vi "remove channel mappings.vi"(8 "error in (no error)":errorcluster, 9 "Properties:UID":string, 10 "Channel Array":refnum<class "TBM channel.lvclass">[](array[class]), 11 "engine configuration in":refnum<class "engine configuration.lvclass">) -> (0 "error out":errorcluster, 1 "Numeric":i32, 2 "Array":string[](array[string]), 3 "engine configuration out":refnum<class "engine configuration.lvclass">, 4 "name":string, 5 "accessors:metadata":string)   [LabVIEW 2015, in "DAQmx Module editor node.lvclass"]
doc: "This VI was createde to encapsulate the multi-channel clearing of mappings on a line during configuration. \n\nThis VI became complicated when we moved to support multiple channels per line. \nWe are trying to minimize code complexity by packaging this mapping cleaning into\nthis subVI."
uses:
  DAQmx Module editor node.lvclass
  <vilib>/NI/Module Execution Interface/Engine Configuration/engine configuration.lvclass
  <vilib>/NI/Tag Bus/tag/tag descriptor.lvclass
  <vilib>/NI/Tag Bus Module Framework/channel/TBM channel.lvclass
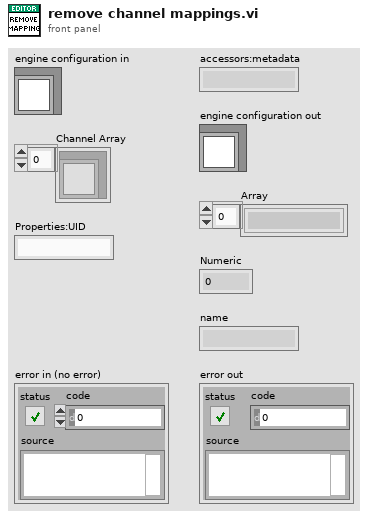
[diagram p1: front panel]
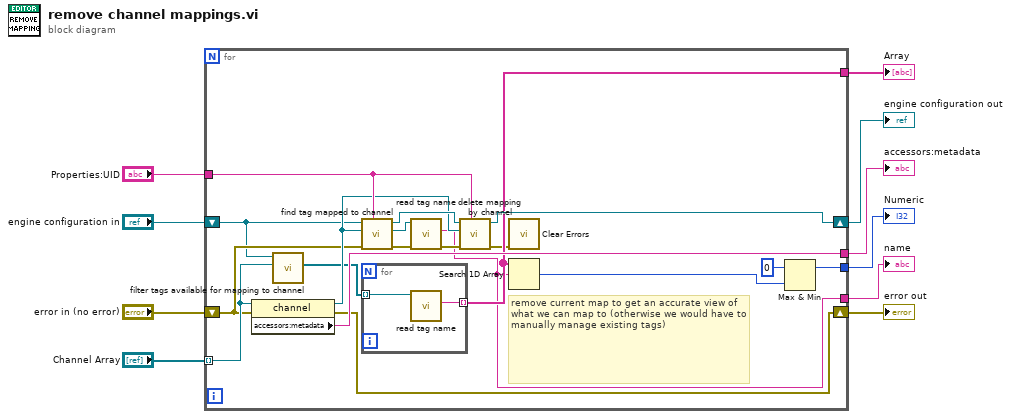
[diagram p0: block diagram]
diagram:
  n1 = for {
    tunnel: [w28] -> w2
    tunnel: "Properties:UID" -> [w27]
    tunnel: "Channel Array" -> [w19] mode=indexing
    tunnel: [w18] -> w6
    tunnel: [w14] -> w7
    tunnel: [w13] -> w8
    shift-right: [w25] -> w4
    shift-left: "error in (no error)" -> [w12]
    shift-right: [w29] -> w1
    shift-left: "engine configuration in" -> [w11]
    # "remove current map to get an accurate view of what we can map to (otherwise we would have to manually manage existing tags)"
    n2 = property class="channel"(reference=w19, error in=w12) -> (reference out=w24:refnum<class "TBM channel.lvclass">, error out=w25:errorcluster, "accessors:metadata"=w28:string)
    n3 = call-dynamic "filter tags available for mapping to channel.vi"("channel to map to"=w19, "engine configuration in"=w11) -> ("filtered tags"=w20:refnum<class "tag descriptor.lvclass">[])  [unwired: 8 in, 1 out]
    n4 = call <vilib>:"find tag mapped to channel.vi"("owner"=w27, "error in"=w12, "channel"=w24, "engine configuration in"=w11) -> ("error out"=w22:errorcluster, "tag"=w23:refnum<class "tag descriptor.lvclass">, "engine configuration out"=w26:refnum<class "engine configuration.lvclass">)  [unwired: 5 in]
    n5 = for {
      tunnel: w20 -> [w31] mode=indexing
      tunnel: [w30] -> w18 mode=indexing
      n6 = call <vilib>:"read tag name.vi"("system tag in"=w31) -> ("name"=w30:string)  [unwired: 8 in, 2 out]
    }
    n7 = call <vilib>:"read tag name.vi"("error in"=w22, "system tag in"=w23) -> ("error out"=w21:errorcluster, "name"=w14:string)  [unwired: 7 in, 1 out]
    n8 = call <vilib>:"delete mapping by channel.vi"("owner ID"=w27, "error in"=w21, "channel"=w24, "engine configuration in"=w26) -> ("error out"=w17:errorcluster, "engine configuration out"=w29:refnum<class "engine configuration.lvclass">)  [unwired: 6 in]
    n9 = call <vilib>:"Clear Errors.vi"("error in (no error)"=w17) -> ()  [unwired: 5 in, 2 out]
    n10 = Search 1D Array(1D array=w18, element=w14) -> (index of element=w15:i32)  [unwired: 1 in]
    n11 = Max & Min(x=0 ("f"), y=w15) -> (max(x,y)=w13:i32)  [unwired: 1 out]
  }
  "Numeric" <- w8
  "name" <- w7
  "Array" <- w6
  "error out" <- w4
  "accessors:metadata" <- w2
  "engine configuration out" <- w1
